vi "Rotate to Vector.vi"(6 "eigen assenstelsel":dbl[](array[numeric])=[-1.0, 1.0, -1.0], 8 "error in (no error)":errorcluster, 9 "Original orient vector":dbl[](array[numeric])=[0.0, 0.0, 1.0], 10 "input vector":dbl[](array[numeric])=[0.0, 0.0, 1.0], 11 "Scene Object":refnum<vi>) -> (0 "error out":errorcluster, 1 "Axis":cluster{"X":sgl, "Y":sgl, "Z":sgl}, 2 "arccos(x)":dbl, 3 "Rotated Scene Object":refnum<vi>)   [LabVIEW 2021]
uses:
  <vilib>/Analysis/baseanly.llb/Real Dot Product.vi
  <vilib>/Analysis/NI_AALPro.lvlib
  <vilib>/Analysis/NI_AALBase.lvlib
  <vilib>/picture/3D Picture Control/NI_3D Picture Control.lvlib
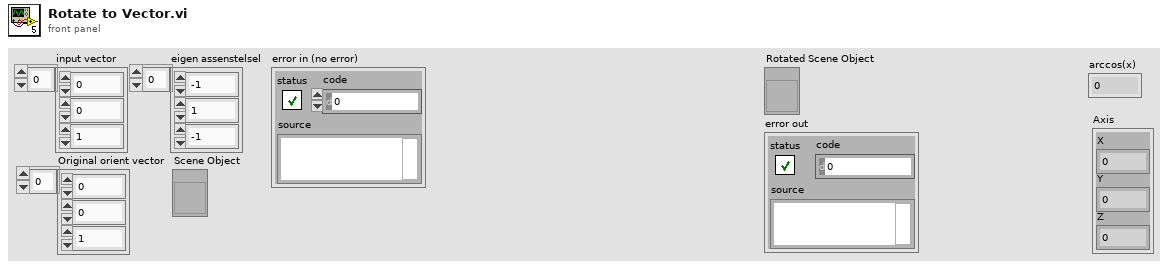
[diagram p1: front panel]
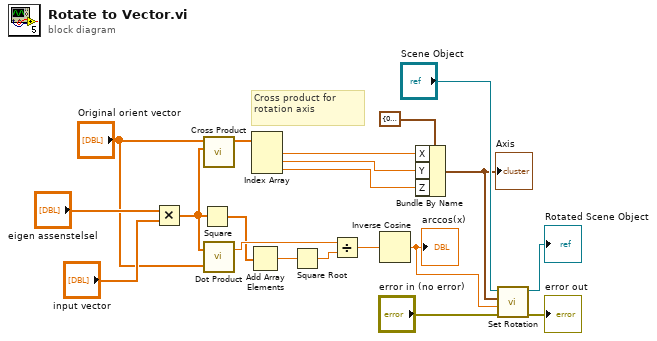
[diagram p0: block diagram]
diagram:
  # "Cross product for rotation axis"
  n1 = Multiply(x="eigen assenstelsel", y="input vector") -> (x*y=w3:dbl[])
  n2 = Square(x=w3) -> (x^2=w10:dbl[])
  n3 = call <vilib>:"Cross Product.vi"("B Vector"=w3, "A Vector"="Original orient vector") -> ("Cross Product"=w19:dbl[])  [unwired: 8 in, 1 out]
  n4 = call-poly <vilib>:"Dot Product.vi"("Y Vector"="Original orient vector", "X Vector"=w3) -> ("X * Y"=w14:dbl)  [unwired: 1 out]
  n5 = Add Array Elements(numeric array=w10) -> (sum=w9:dbl)
  n6 = Index Array(array=w19) -> (element #1=w16:dbl, element #2=w17:dbl, element #3=w18:dbl)  [unwired: 3 in]
  n7 = Square Root(x=w9) -> (sqrt(x)=w20:dbl)
  n8 = Divide(x=w14, y=w20) -> (x/y=w15:dbl)
  n9 = Inverse Cosine(1:w15) -> (0:w12:dbl)
  "arccos(x)" <- w12
  n10 = Bundle By Name(cluster=cluster{"X":sgl, "Y":sgl, "Z":sgl} {"X"=0.0, "Y"=0.0, "Z"=0.0} ("Translation"), "X"=w16, "Y"=w17, "Z"=w18) -> (w4:cluster{"X":sgl, "Y":sgl, "Z":sgl})
  "Axis" <- w4
  n11 = call <vilib>:"Set Rotation.vi"("error in (no error)"="error in (no error)", "Angle"=w12, "Axis"=w4, "Scene Object"="Scene Object") -> ("error out"=→"error out":errorcluster, "Rotated Scene Object"=→"Rotated Scene Object":refnum<vi>)  [unwired: 6 in]
